vi "LakeShore 336 Get Curve Header Info.vi"(2 "Curve #":i32, 3 "VISA session":refnum<visa-resource-name>) -> (0 "Cluster":T2 {"Temp. Coef" items=["????", "Negative", "Positive"]; "Setpoint Limit" format="%.4f"; "Data Format" items=["mV/K"=1, "V/K"=2, "½/K"=3, "Log ½/K"=4]}, 1 "dup VISA session":refnum<visa-resource-name>)   [LabVIEW 2019]
doc: "This VI reads a curve header from the LakeShore Model 370 AC Resistance Bridge and returns the parsed data.\nScott Hannahs, <sth@magnet.fsu.edu> NHMFL-FSU, May 2003"
uses:
  Misc Extras/Manufacturer Drivers/LakeShore/Lake Shore Cryotronics 336/Public/Utility/Data Format.ctl
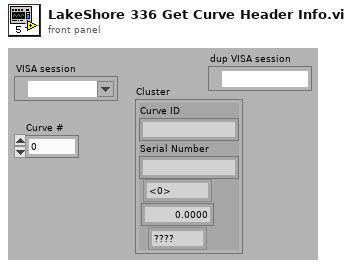
[diagram p1: front panel]
types:
  T1 = typedef "Data Format.ctl" = u16
  T2 = cluster{"Curve ID":string, "Serial Number":string, "Data Format":T1, "Setpoint Limit":dbl, "Temp. Coef":u16}
  T3 = cluster{"String Returned":string, "String Returned":string, i32, dbl, i32}
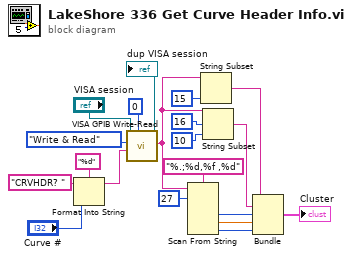
[diagram p0: block diagram]
diagram:
  n1 = Format Into String(format string="%d", initial string="CRVHDR? " ("String to Write"), "Curve #") -> (resulting string=w8:string)  [unwired: 1 in, 1 out]
  n2 = call "VISA GPIB Write-Read.vi"("Wait (ms)"=u32 0 ("wait (mS)"), "Command"=w8, "Action"=enum16{"Write", "Read", "Write & Read"}."Write & Read", "VISA resource name"="VISA session") -> ("String Returned"=w19:string, "dup VISA Session"=→"dup VISA session":refnum<visa-resource-name>)  [unwired: 4 in, 2 out]
  n3 = Scan From String(format string="%.;%d,%f ,%d", input string=w19, initial scan location=u32 27) -> (output 1=w10:i32, output 2=w11:dbl, output 3=w12:i32)  [unwired: 4 in, 3 out]
  n4 = String Subset(string=w19, length (rest)=15 ("length (rest)")) -> (substring=w18:string)  [unwired: 1 in]
  n5 = String Subset(string=w19, offset (0)=16, length (rest)=10 ("offset (0)")) -> (substring=w17:string)
  n6 = Bundle("String Returned"=w18, "String Returned"=w17, w10, w11, w12) -> (→"Cluster":T3)  [unwired: 1 in]
